vi "Fail If Specific Error.vi"(6 "Error Codes":i32[](array[numeric]), 7 "Description":string, 8 "error in (no error)":errorcluster, 10 "Assert error":errorcluster, 11 "LUnit Test Case In":refnum<class "LUnit Test Case.lvclass">) -> (0 "error out":errorcluster, 3 "LUnit Test Case Out":refnum<class "LUnit Test Case.lvclass">)   [LabVIEW 2020, in "Advanced Assertions.lvlib"]
doc: "Generates a fail result for the calling test method if the inputs contains an error with status \"True\". Using the Error Codes input it is possible to select which specific error codes to test for. A description may be provided to the result."
uses:
  Advanced Assertions.lvlib
  LUnit Test Case/LUnit Test Case.lvclass
  LUnit Test Case/LUnit Test Case.lvclass/LUnit Test Case.ctl
  c764aba1-6191-4a45-99b6-9f14aa7c11f7.vi
  LUnit Test Case/Private/Append Pass Result.vi
  LUnit Test Case/Private/Append Fail Result.vi
  <vilib>/Comparison/Equal/Equal Functor/Equal Functor.lvclass
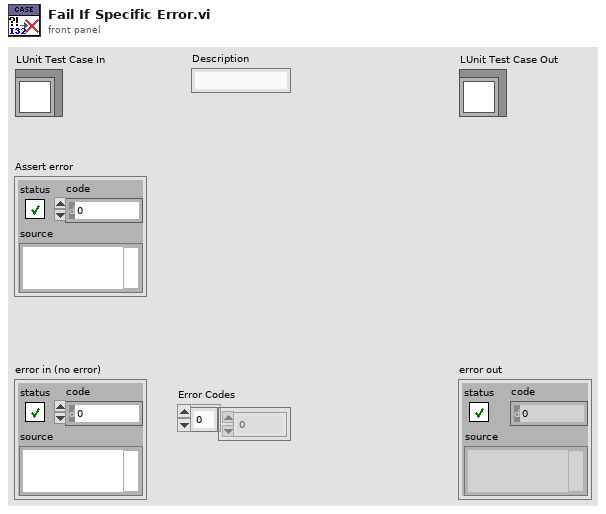
[diagram p1: front panel]
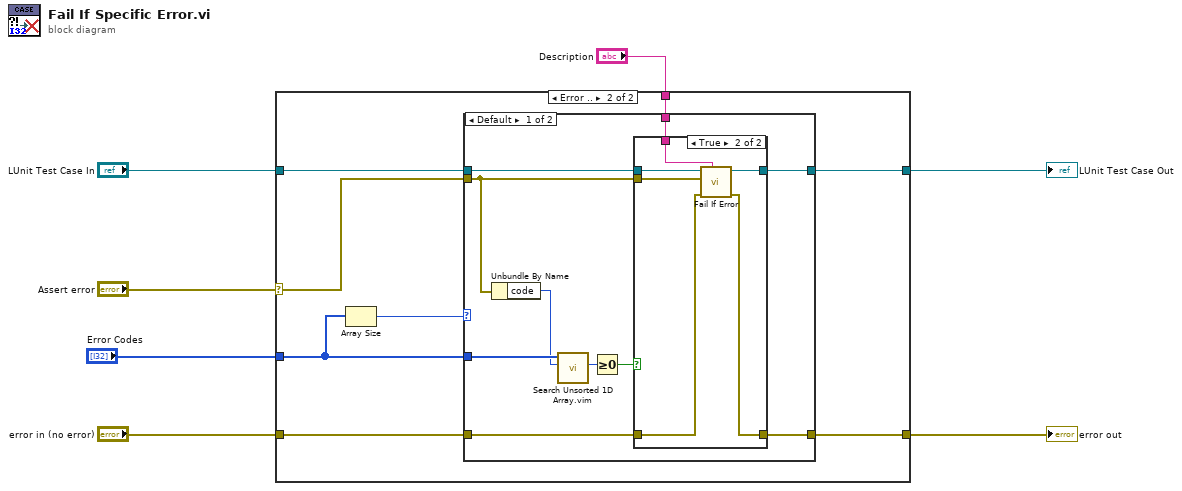
[diagram p0: block diagram]
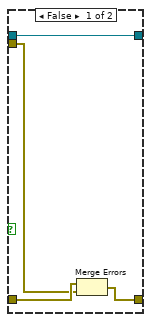
[diagram p3: hidden frame]
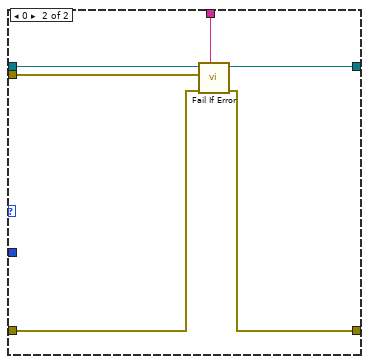
[diagram p4: hidden frame]
diagram:
  n1 = case shown="Error .." "Assert error" {
    selector: "Assert error" -> [_ w13]
    tunnel: "LUnit Test Case In" -> [w9 w17]
    tunnel: [w9 w16] -> w5
    tunnel: [w8 w15] -> w4
    tunnel: "Description" -> [_ w12]
    tunnel: "error in (no error)" -> [w8 w14]
    tunnel: "Error Codes" -> [_ w10]
    frame No Error {
    }
    frame Error {
      n2 = Array Size(array=w10) -> (size(s)=w11:i32)
      n3 = case shown="Default" w11 {
        tunnel: w17 -> [w27 w43]
        tunnel: [w24 w42] -> w16
        tunnel: [w25 w41] -> w15
        tunnel: w14 -> [w26 w40]
        tunnel: w13 -> [w19 w39]
        tunnel: w12 -> [w23 w38]
        tunnel: w10 -> [w22 _]
        frame Default {
          n4 = Unbundle By Name(w19) -> ("code"=w18:i32)
          n5 = call "Search Unsorted 1D Array.vim"("element"=w18, "unsorted 1D array"=w22) -> ("index of element"=w21:i32)  [unwired: 9 in]
          n6 = Greater Or Equal To 0?(x=w21) -> (x >= 0?=w20:bool)
          n7 = case shown="True" w20 {
            tunnel: w27 -> [w31 w37]
            tunnel: w19 -> [w28 w36]
            tunnel: w26 -> [w29 w35]
            tunnel: [w30 w34] -> w25
            tunnel: [w31 w33] -> w24
            tunnel: w23 -> [_ w32]
            frame False {
              n8 = Merge Errors(w29, w28) -> (w30:errorcluster)
            }
            frame True {
              n9 = call "Fail If Error.vi"("Description"=w32, "error in (no error)"=w35, "Assert error"=w36, "LUnit Test Case In"=w37) -> ("error out"=w34:errorcluster, "LUnit Test Case Out"=w33:refnum<class "LUnit Test Case.lvclass">)  [unwired: 6 in]
            }
          }
        }
        frame 0 {
          n10 = call "Fail If Error.vi"("Description"=w38, "error in (no error)"=w40, "Assert error"=w39, "LUnit Test Case In"=w43) -> ("error out"=w41:errorcluster, "LUnit Test Case Out"=w42:refnum<class "LUnit Test Case.lvclass">)  [unwired: 6 in]
        }
      }
    }
  }
  "error out" <- w4
  "LUnit Test Case Out" <- w5
